vi "Server 2 - Copy.vi"() -> ()   [LabVIEW 2017]
uses:
  <vilib>/Analysis/Matrix/Datatypes/RealMatrix.ctl
  <vilib>/Analysis/Matrix/NI_Matrix.lvlib
panel:
  out "array":dbl[](array[numeric])
  out "number 2":dbl
  out "substring":string
  out "number":dbl
  out "M1 x M2 2":T1
  out "data out":string
  in  "stop":bool
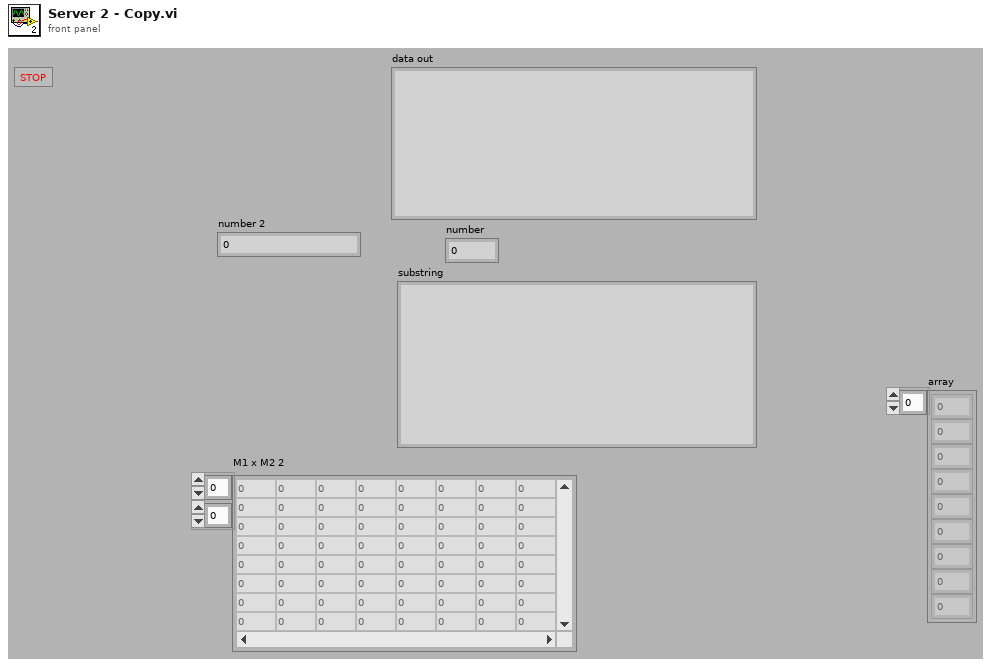
[diagram p1: front panel]
types:
  T1 = typedef "NI_Matrix.lvlib/RealMatrix.ctl" = dbl[][]
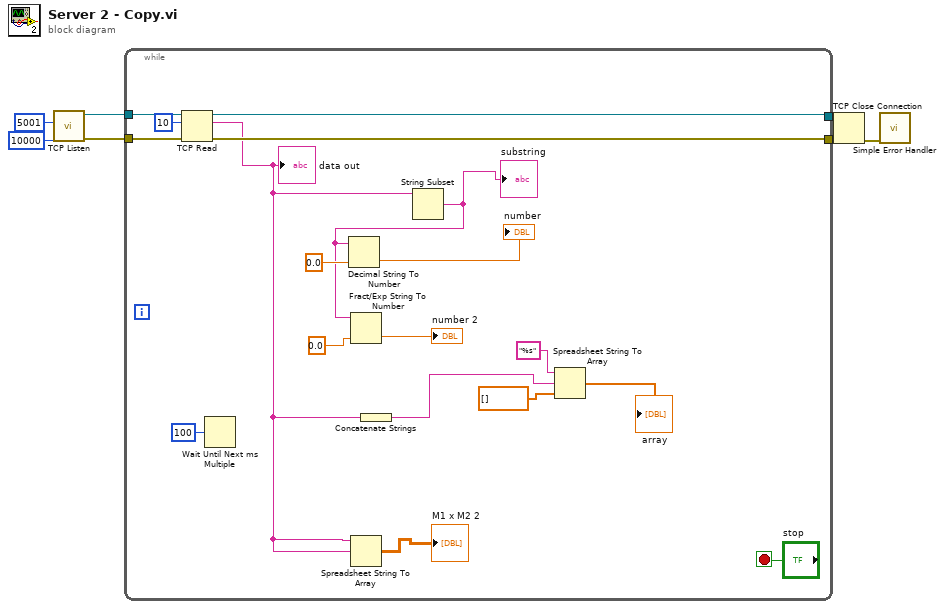
[diagram p0: block diagram]
diagram:
  n1 = call <vilib>:"TCP Listen.vi"("timeout ms (wait forever: -1)"=10000, "port"=u16 5001) -> ("error out"=w6:errorcluster, "connection ID"=w7:refnum<k5>)  [unwired: 5 in, 3 out]
  n2 = while {
    tunnel: w7 -> [w24]
    tunnel: w6 -> [w23]
    tunnel: [w20] -> w5
    tunnel: [w22] -> w4
    stop <- "stop" stop-if-true
    n3 = TCP Read(connection ID=w24, bytes to read=10, error in (no error)=w23) -> (connection ID out=w20:refnum<k5>, data out=w8:string, error out=w22:errorcluster)  [unwired: 2 in]
    "data out" <- w8
    n4 = Wait Until Next ms Multiple(millisecond multiple=u32 100) -> ()  [unwired: 1 out]
    n5 = Spreadsheet String To Array(format string=w8, spreadsheet string=w8) -> (array=→"M1 x M2 2":dbl[][])  [unwired: 2 in]
    n6 = Concatenate Strings(w8) -> (w12:string)
    n7 = String Subset(string=w8) -> (substring=w15:string)  [unwired: 2 in]
    "substring" <- w15
    n8 = Decimal String To Number(string=w15, default (0L)=0.0 ("y")) -> (number=→"number":dbl)  [unwired: 1 in, 1 out]
    n9 = Fract/Exp String To Number(string=w15, default (0 dbl)=0.0 ("y")) -> (number=→"number 2":dbl)  [unwired: 2 in, 1 out]
    n10 = Spreadsheet String To Array(format string="%s", spreadsheet string=w12, array type (2D Dbl)=dbl[] []) -> (array=→"array":dbl[])  [unwired: 1 in]
  }
  n11 = TCP Close Connection(connection ID=w5, error in (no error)=w4) -> (error out=w3:errorcluster)  [unwired: 1 in, 1 out]
  n12 = call <vilib>:"Simple Error Handler.vi"("error in (no error)"=w3) -> ()  [unwired: 4 in, 5 out]
